vi "Make Short Class Name.vi"(11 "Class Name":string) -> (3 "Shortened Class Name":string)   [LabVIEW 2020, in "NI_VIAnCFGDataStructure.lvlib" / "Tree.lvclass"]
uses:
  <vilib>/addons/analyzer/VIAnCFGDataStructure/Tree Manager/Tree.lvclass
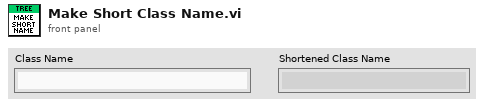
[diagram p1: front panel]
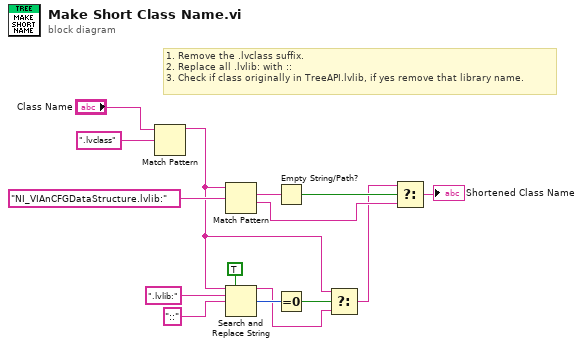
[diagram p0: block diagram]
diagram:
  # "1. Remove the .lvclass suffix.\n2. Replace all .lvlib: with ::\n3. Check if class originally in TreeAPI.lvlib, if yes remove that library name."
  n1 = Match Pattern(string="Class Name", regular expression=".lvclass") -> (before substring=w2:string)  [unwired: 1 in, 3 out]
  n2 = Match Pattern(string=w2, regular expression="NI_VIAnCFGDataStructure.lvlib:") -> (match substring=w12:string, after substring=w14:string)  [unwired: 1 in, 2 out]
  n3 = Search and Replace String(replace all?=TRUE ("replace all? (F)"), input string=w2, search string=".lvlib:" ("regular expression"), replace string="::" ("replace string (\"\")")) -> (result string=w3:string, number of replacements=w5:i32)  [unwired: 4 in, 2 out]
  n4 = Empty String/Path?(string/path=w12) -> (empty?=w13:bool)
  n5 = Equal To 0?(x=w5) -> (x = 0?=w4:bool)
  n6 = Select(t=w2, s=w4, f=w3) -> (s? t:f=w1:string)
  n7 = Select(t=w1, s=w13, f=w14) -> (s? t:f=→"Shortened Class Name":string)
